vi "16 pulses TX.vi"(7 "reset system clock":bool, 10 "input Valid":bool, 11 "array PDW":u64[](array[numeric])=[0, 0, 0, 0, 0, 0, 0, 0]) -> (0 "pulse transmitted":u32, 1 "fpga clock":u64, 2 "dds free":bool[](array[boolean]), 3 "RF OUT":T1, 4 "ready for input":bool)   [LabVIEW 2021]
uses:
  <instrlib>/_niInstr/DSP/v1/Shared/Public/IQ Data.ctl
  <instrlib>/_niInstr/Basic Elements/v1/FPGA/Private/Count Up U64.vi
  <instrlib>/_niInstr/Basic Elements/v1/FPGA/Private/Count Up U32.vi
  <instrlib>/_niInstr/Basic Elements/v1/FPGA/niInstr Basic Elements v1 FPGA.lvlib
  <instrlib>/_niInstr/DSP/v1/Shared/niInstr DSP v1 Shared.lvlib
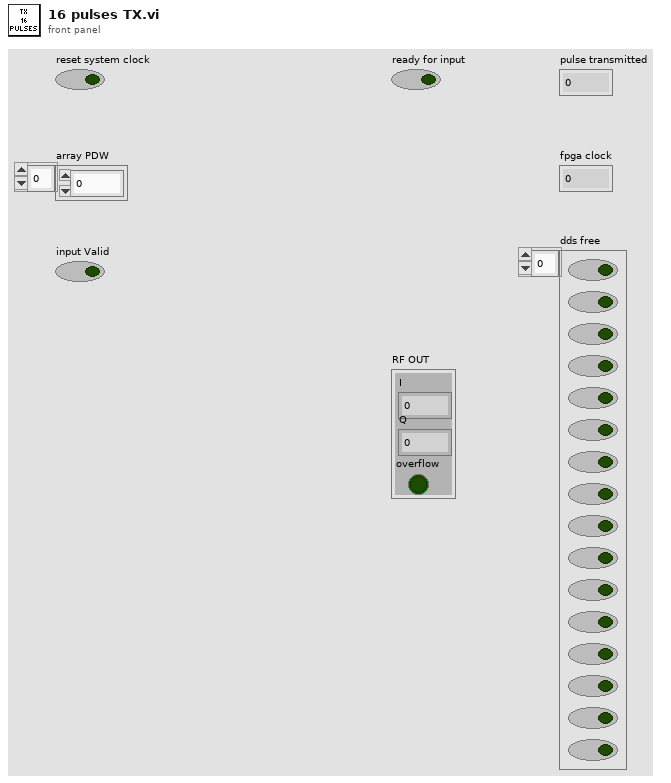
[diagram p1: front panel]
types:
  T1 = typedef "niInstr DSP v1 Shared.lvlib/IQ Data.ctl" = cluster{"I":fxp<+/-,18,1>, "Q":fxp<+/-,18,1>, "overflow":bool}
  T2 = typedef "pdw.ctl" = cluster{"PW":u32, "frequency shift":fxp<+/-,48,0>, "amp":fxp<+/-,18,1>, "mode type":u8, "mode file":u8, "mode depth":u32, "filter rate_pulse":u16, "filter rate bpsk":u16}
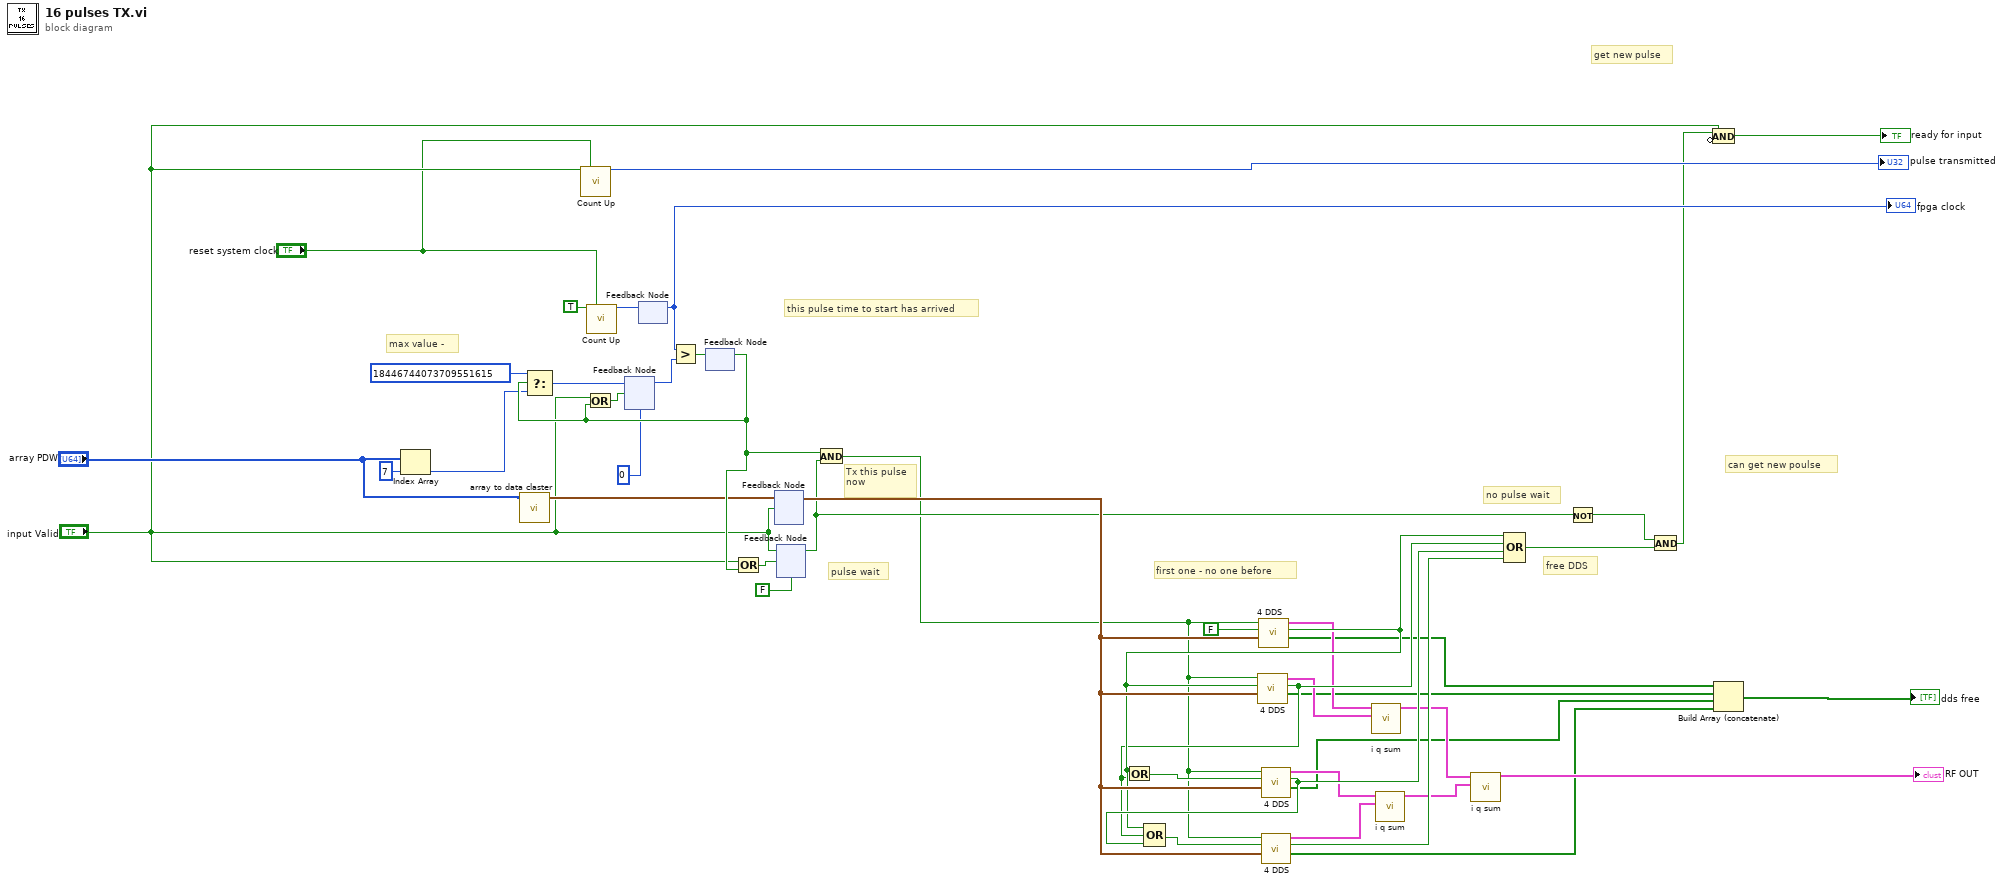
[diagram p0: block diagram]
diagram:
  # "this pulse time to start has arrived"
  # "first one - no one before"
  # "max value -"
  # "Tx this pulse\nnow"
  # "get new pulse"
  # "pulse wait"
  # "can get new poulse"
  # "no pulse wait"
  # "free DDS"
  n1 = Index Array(array="array PDW", index=7) -> (element=w41:u64)
  n2 = call "array to data claster.vi"("Array"="array PDW") -> ("Cluster"=w22:T2)  [unwired: 10 in]
  n3 = call-poly <instrlib>:"Count Up.vi"("increment"="input Valid", "reset"="reset system clock") -> ("count out"=→"pulse transmitted":u32)  [unwired: 13 in]
  n4 = call-poly <instrlib>:"Count Up.vi"("increment"=TRUE, "reset"="reset system clock") -> ("count out"=w20:u64)  [unwired: 13 in]
  n5 = feedback #1(u64 0 ("U64")) -> (w7:u64)
  n6 = feedback #2() -> (w21:u64)  [unwired: 1 in]
  "fpga clock" <- w21
  n7 = feedback-in #2(w20) -> ()
  n8 = Greater?(x=w21, y=w7) -> (0:w44:bool)
  n9 = feedback #3() -> (w45:bool)  [unwired: 1 in]
  n10 = Select(t=u64 18446744073709551615, s=w45, f=w41) -> (s? t:f=w12:u64)
  n11 = Or(x="input Valid", y=w45) -> (x .or. y?=w13:bool)
  n12 = feedback-in #1(w12, w13) -> ()
  n13 = feedback-in #3(w44) -> ()
  n14 = Or(x="input Valid", y=w45) -> (x .or. y?=w18:bool)
  n15 = feedback #4() -> (w38:T2)  [unwired: 1 in]
  n16 = feedback-in #4(w22, "input Valid") -> ()
  n17 = feedback #5(FALSE ("Output Valid")) -> (w30:bool)
  n18 = feedback-in #5("input Valid", w18) -> ()
  n19 = And(x=w45, y=w30) -> (x .and. y?=w5:bool)
  n20 = call "4 DDS.vi"("pdw in"=w38, "free DDS before me?"=FALSE, "new PDW in"=w5) -> ("state of every DDS"=w4:bool[], "have free DDS"=w36:bool, "IQ out"=w29:T1)  [unwired: 6 in]
  n21 = call "4 DDS.vi"("pdw in"=w38, "free DDS before me?"=w36, "new PDW in"=w5) -> ("state of every DDS"=w3:bool[], "have free DDS"=w35:bool, "IQ out"=w31:T1)  [unwired: 6 in]
  n22 = Or(x=w36, y=w35) -> (x .or. y?=w32:bool)
  n23 = call "4 DDS.vi"("pdw in"=w38, "free DDS before me?"=w32, "new PDW in"=w5) -> ("state of every DDS"=w2:bool[], "have free DDS"=w39:bool, "IQ out"=w33:T1)  [unwired: 6 in]
  n24 = Compound Arithmetic op=OR(w36, w35, w39) -> (w37:bool)
  n25 = call "4 DDS.vi"("pdw in"=w38, "free DDS before me?"=w37, "new PDW in"=w5) -> ("state of every DDS"=w1:bool[], "have free DDS"=w40:bool, "IQ out"=w34:T1)  [unwired: 6 in]
  n26 = call "i q sum.vi"(10:"data in"=w31, 11:"data in"=w29) -> ("output cluster"=w25:T1)  [unwired: 9 in]
  n27 = call "i q sum.vi"(10:"data in"=w34, 11:"data in"=w33) -> ("output cluster"=w27:T1)  [unwired: 9 in]
  n28 = call "i q sum.vi"(10:"data in"=w27, 11:"data in"=w25) -> ("output cluster"=→"RF OUT":T1)  [unwired: 9 in]
  n29 = Compound Arithmetic op=OR(w36, w35, w39, w40) -> (w23:bool)
  n30 = Not(x=w30) -> (.not. x?=w8:bool)
  n31 = And(x=w8, y=w23) -> (x .and. y?=w9:bool)
  n32 = Compound Arithmetic op=AND(w9, invert "input Valid") -> (→"ready for input":bool)
  n33 = Build Array (concatenate)(w4, w3, w2, w1) -> (→"dds free":bool[])
